vi "init Font.vi"(8 "error in (no error)":errorcluster, 11 "ScintillaNET in":refnum<class "ScintillaNET.lvclass">) -> (0 "error out":errorcluster, 3 "ScintillaNET out":refnum<class "ScintillaNET.lvclass">)   [LabVIEW 2018, in "ScintillaNET.lvclass"]
uses:
  ScintillaNET.lvclass
  D:/project/hobby/LF2R/LabVIEW/source/ScintillaNET/dll/ScintillaNET.dll
  dll/ScintillaNET.dll
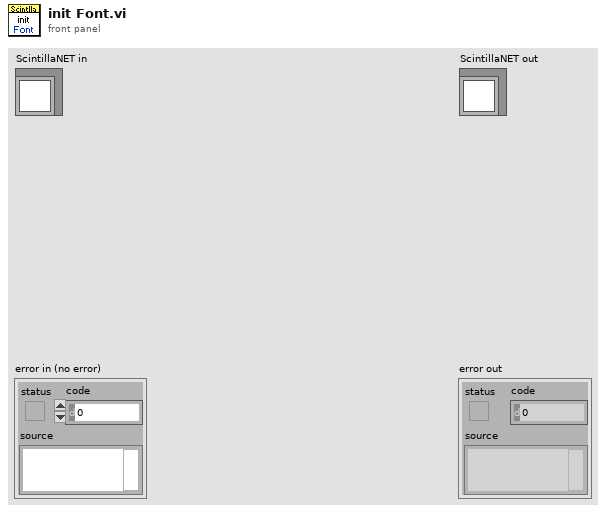
[diagram p1: front panel]
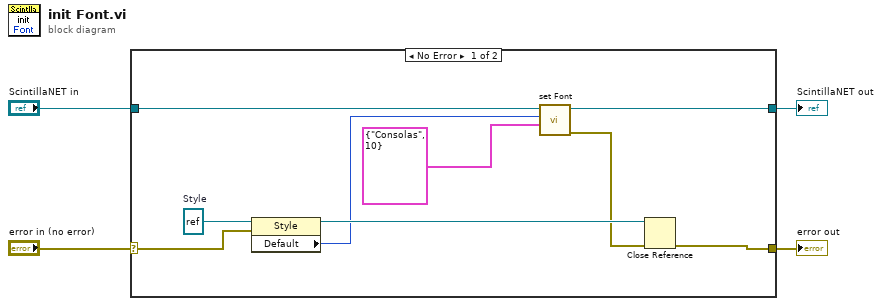
[diagram p0: block diagram]
diagram:
  n1 = case shown="No Error" "error in (no error)" {
    selector: "error in (no error)" -> [w12 w15]
    tunnel: [w11 w15] -> w3
    tunnel: [w8 w14] -> w1
    tunnel: "ScintillaNET in" -> [w9 w14]
    frame No Error {
      w13 = refnum<k24> refnum  # Style
      n2 = property class="Style"(reference=w13, error in=w12) -> (reference out=w10:refnum<k24>, "Default"=w6:i32)  [unwired: 1 out]
      n3 = call "set Font.vi"("Font"=cluster{"Font":string, "Size":i32} {"Font"="Consolas", "Size"=10}, "Style index"=w6, "ScintillaNET in"=w9) -> ("error out"=w7:errorcluster, "ScintillaNET out"=w8:refnum<class "ScintillaNET.lvclass">)  [unwired: 7 in]
      n4 = Close Reference(reference=w10, error in (no error)=w7) -> (error out=w11:errorcluster)
    }
    frame Error {
    }
  }
  "error out" <- w3
  "ScintillaNET out" <- w1
